vi "Demo - Simple Use.vi"() -> ()   [LabVIEW 2020, in "GOLPI library.lvlib"]
doc: "Very simple demonstration of use of the GOLPI library.\n\n---\nGOLPI works only with lv_proc.dll library, which is part of vipm package or should be delivered together with packed library. Placement of this dll is selected in terminal of Start GNU Octave.vi."
uses:
  GOLPI library.lvlib
panel:
  in  "octave exe file or directory":path=path "C:/Octave/Octave-4.0.0/bin"
  in  "command":string="sin(3)"
  out "GNU Octave version":string
  out "exit code":i32
  out "error out":errorcluster
  out "read buffer":string
  in  "working directory":path=path "C:/"
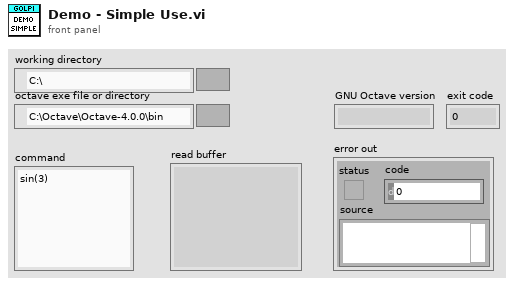
[diagram p1: front panel]
types:
  T1 = typedef "GOLPI library.lvlib/GOLPI reference Type Def.ctl" = cluster{"pipe handle":T2, "fast read timeout [ms]":u32, "fast read settle time [ms]":u32, "fast read to multiple [ms]":u32, "max elements per input line":u32, "slow read timeout [ms]":u32, "stdin double format specifier":string, "max elements per stdout output column":u32, "console mode bitstream":bool, "bitstream first read timeout [ms]":u32, "bitstream read timeout [ms]":u32, "struct transfer possible":bool, "matlab mode":bool}
  T2 = typedef "LV Process library.lvlib/Pipe Handle.ctl" = cluster{"lv_proc.dll file path":path, "process instance handle":u32[], "debug mode":bool, "debug data":cluster{"time":timestamp, "stdin":bool, "data":string}[]}
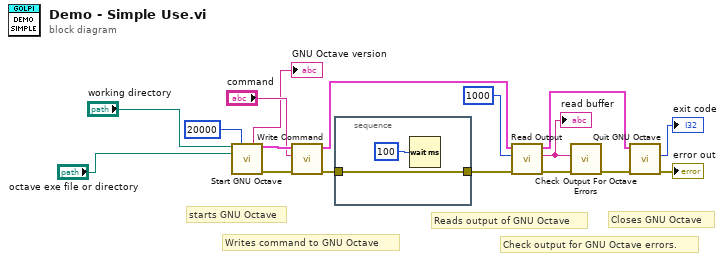
[diagram p0: block diagram]
diagram:
  # "Check output for GNU Octave errors."
  # "Closes GNU Octave"
  # "Reads output of GNU Octave"
  # "Writes command to GNU Octave"
  # "starts GNU Octave"
  n1 = call "Start GNU Octave.vi"("working dir (user home)"="working directory", "full start timeout [ms] (20000)"=u32 20000 ("Full start timeout [ms] (5000)"), "octave binary file or dir (autofind)"="octave exe file or directory") -> ("GNU Octave version"=→"GNU Octave version":string, "GOLPI ref. out"=w16:T1, "error out"=w13:errorcluster)  [unwired: 9 in, 1 out]
  n2 = call "Write Command.vi"("error in"=w13, "command"="command", "GOLPI ref. in"=w16) -> ("error out"=w12:errorcluster, "GOLPI ref. out"=w15:T1)  [unwired: 7 in]
  n3 = stacked-sequence {
    tunnel: [w18] -> w11
    tunnel: w12 -> [w18]
    frame #0 {
      n4 = Wait (ms)(milliseconds to wait=u32 100) -> ()  [unwired: 1 out]
    }
  }
  n5 = call "Read Output.vi"("error in"=w11, "byte count"=1000, "GOLPI ref. in"=w15) -> ("error out"=w3:errorcluster, "read buffer"=w4:string, "GOLPI ref. out"=w14:T1)  [unwired: 5 in, 1 out]
  "read buffer" <- w4
  n6 = call "Check Output For Octave Errors.vi"("error in"=w3, "read buffer"=w4) -> ("error out"=w2:errorcluster)  [unwired: 9 in]
  n7 = call "Quit GNU Octave.vi"("error in"=w2, "GOLPI ref. in"=w14) -> ("error out"=→"error out":errorcluster, "exit code"=→"exit code":i32)  [unwired: 8 in]
